vi "FgenChannelData2 FPCluster.vi"(8 "error in (no error)":errorcluster, 10 "Channel Index":i32, 11 "CS++FgenChannelData in":refnum<class "CS++FgenChannelData.lvclass">) -> (0 "error out":errorcluster, 1 "FM-Modulation":cluster{"Enabled":bool, "Source":i32}={"Enabled"=TRUE, "Source"=0} {"Source" items=["Internal", "External"]}, 2 "AM-Modulation":cluster{"Enabled":bool, "Source":i32}={"Enabled"=TRUE, "Source"=0} {"Source" items=["Internal", "External"]}, 3 "Standard-Waveform":T2={"Enabled"=TRUE, "Operation Mode"=0, "Impedance"=50.0, "Waveform"=1, "Frequency"=1000.0, "Amplitude"=1.0, "DC Offset"=0.0, "Trigger Source"=1, "Burst Count"=1, "Start Phase"=0.0, "Set/Single"=FALSE} {"Start Phase" format="%.3f"; "Trigger Source" items=["Internal"=3, "External"=1, "Software Trigger Function"=2, "PXI TRIG0 or VXI TTL0"=111, "PXI TRIG1 or VXI TTL1"=112, "PXI TRIG2 or VXI TTL2"=113, "PXI TRIG3 or VXI TTL3"=114, "PXI TRIG4 or VXI TTL4"=115, "PXI TRIG5 or VXI TTL5"=116, "PXI TRIG6 or VXI TTL6"=117, "PXI TRIG7 or VXI TTL7"=118, "ECL0"=119, "ECL1"=120, "PXI Star"=131, "RTSI 0"=141, "RTSI 1"=142, "RTSI 2"=143, "RTSI 3"=144, "RTSI 4"=145, "RTSI 5"=146, "RTSI 6"=147]; "Frequency" format="%^.3e"; "DC Offset" format="%.3f"; "Amplitude" format="%.3f"; "Waveform" items=["Sine"=1, "Square"=2, "Triangle"=3, "Ramp Up"=4, "Ramp Down"=5, "DC"=6]; "Impedance" format="%.3f"; "Operation Mode" items=["Continuous", "Burst"]}, 4 "Advanced Trigger":T1 {"Trigger Slope)" items=["Positive", "Negative", "Either"]}, 5 "Resume Trigger":T1 {"Trigger Slope)" items=["Positive", "Negative", "Either"]}, 6 "Stop Trigger":T1 {"Trigger Slope)" items=["Positive", "Negative", "Either"]}, 7 "Start Trigger":T1 {"Trigger Slope)" items=["Positive", "Negative", "Either"]})   [LabVIEW 2013, in "CS++FgenGui.lvlib" / "CS++FgenGui.lvclass"]
doc: "This VI read channel data from object and writes it into FP cluster."
uses:
  CS++FgenGui.lvclass
  CS++FgenChannelData/CS++FgenChannelData.lvclass
  CS++FgenChannelData/CS++FgenChannelData.lvclass/CS++FgenChannelData.ctl
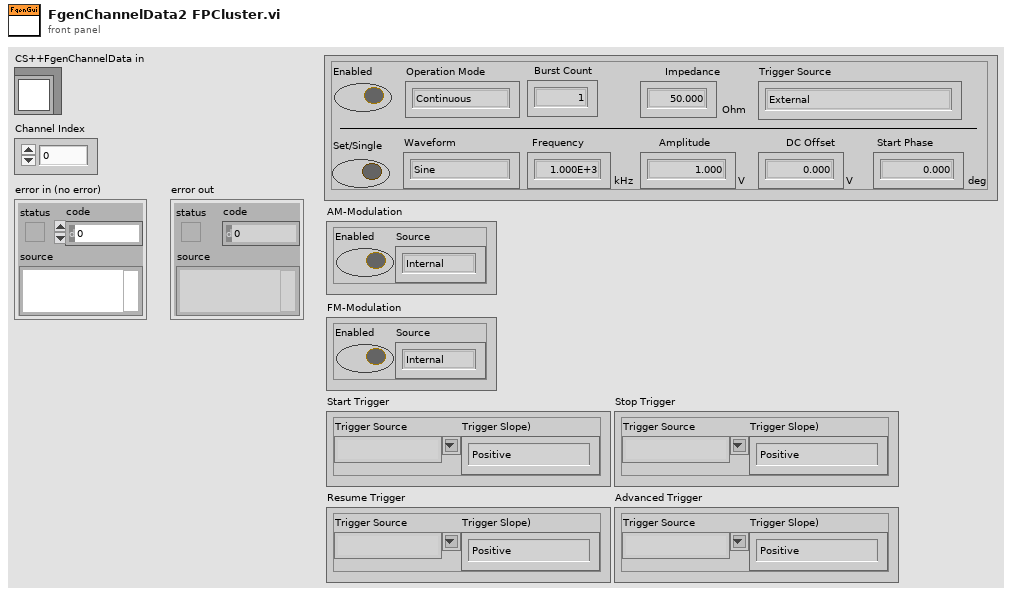
[diagram p1: front panel]
types:
  T1 = cluster{"Trigger Source":string, "Trigger Slope)":i32}
  T2 = cluster{"Enabled":bool, "Operation Mode":i32, "Impedance":dbl[unit], "Waveform":i32, "Frequency":dbl[unit], "Amplitude":dbl[unit], "DC Offset":dbl[unit], "Trigger Source":i32, "Burst Count":i32, "Start Phase":dbl[unit], "Set/Single":bool}
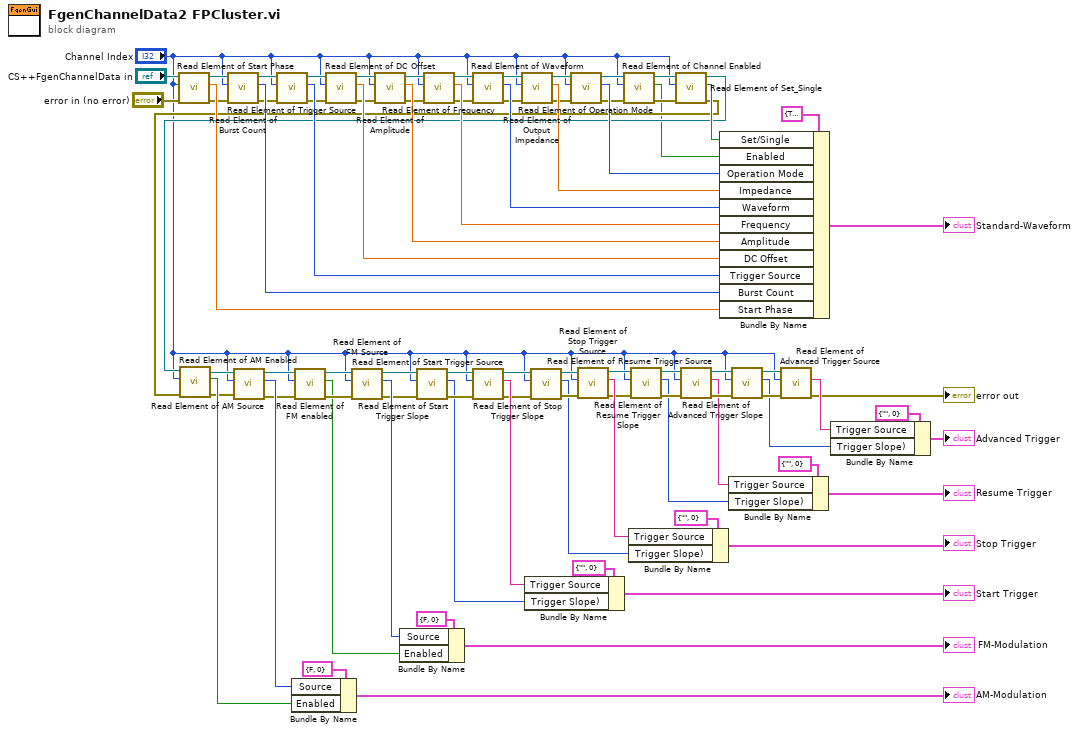
[diagram p0: block diagram]
diagram:
  n1 = call "Read Element of Start Phase.vi"("error in (no error)"="error in (no error)", "index"="Channel Index", "CS++FgenChannelData in"="CS++FgenChannelData in") -> ("error out"=w61:errorcluster, "start phase (0.00 Degrees)"=w71:dbl[unit], "CS++FgenChannelData out"=w69:refnum<class "CS++FgenChannelData.lvclass">)  [unwired: 6 in]
  n2 = call "Read Element of Burst Count.vi"("error in (no error)"=w61, "index"="Channel Index", "CS++FgenChannelData in"=w69) -> ("error out"=w62:errorcluster, "burst count (1)"=w72:i32, "CS++FgenChannelData out"=w70:refnum<class "CS++FgenChannelData.lvclass">)  [unwired: 6 in]
  n3 = call "Read Element of Trigger Source.vi"("error in (no error)"=w62, "index"="Channel Index", "CS++FgenChannelData in"=w70) -> ("error out"=w63:errorcluster, "trigger source (External)"=w73:i32, "CS++FgenChannelData out"=w74:refnum<class "CS++FgenChannelData.lvclass">)  [unwired: 6 in]
  n4 = call "Read Element of DC Offset.vi"("error in (no error)"=w63, "index"="Channel Index", "CS++FgenChannelData in"=w74) -> ("error out"=w64:errorcluster, "dc offset (0.00 V)"=w76:dbl[unit], "CS++FgenChannelData out"=w75:refnum<class "CS++FgenChannelData.lvclass">)  [unwired: 6 in]
  n5 = call "Read Element of Amplitude.vi"("error in (no error)"=w64, "index"="Channel Index", "CS++FgenChannelData in"=w75) -> ("error out"=w65:errorcluster, "amplitude (1.00 V)"=w77:dbl[unit], "CS++FgenChannelData out"=w78:refnum<class "CS++FgenChannelData.lvclass">)  [unwired: 6 in]
  n6 = call "Read Element of Frequency.vi"("error in (no error)"=w65, "index"="Channel Index", "CS++FgenChannelData in"=w78) -> ("error out"=w66:errorcluster, "frequency (1000.0 Hz)"=w79:dbl[unit], "CS++FgenChannelData out"=w80:refnum<class "CS++FgenChannelData.lvclass">)  [unwired: 6 in]
  n7 = call "Read Element of Waveform.vi"("error in (no error)"=w66, "index"="Channel Index", "CS++FgenChannelData in"=w80) -> ("error out"=w67:errorcluster, "waveform (Sine)"=w81:i32, "CS++FgenChannelData out"=w82:refnum<class "CS++FgenChannelData.lvclass">)  [unwired: 6 in]
  n8 = call "Read Element of Output Impedance.vi"("error in (no error)"=w67, "index"="Channel Index", "CS++FgenChannelData in"=w82) -> ("error out"=w68:errorcluster, "impedance (50 Ohms)"=w83:dbl[unit], "CS++FgenChannelData out"=w84:refnum<class "CS++FgenChannelData.lvclass">)  [unwired: 6 in]
  n9 = call "Read Element of Operation Mode.vi"("error in (no error)"=w68, "index"="Channel Index", "CS++FgenChannelData in"=w84) -> ("error out"=w4:errorcluster, "operation mode (Continuous)"=w85:i32, "CS++FgenChannelData out"=w6:refnum<class "CS++FgenChannelData.lvclass">)  [unwired: 6 in]
  n10 = call "Read Element of Channel Enabled.vi"("error in (no error)"=w4, "index"="Channel Index", "CS++FgenChannelData in"=w6) -> ("error out"=w2:errorcluster, "channel enabled (True)"=w1:bool, "CS++FgenChannelData out"=w5:refnum<class "CS++FgenChannelData.lvclass">)  [unwired: 6 in]
  n11 = call "Read Element of Set_Single.vi"("error in (no error)"=w2, "index"="Channel Index", "CS++FgenChannelData in"=w5) -> ("error out"=w8:errorcluster, "Set/Single"=w9:bool, "CS++FgenChannelData out"=w7:refnum<class "CS++FgenChannelData.lvclass">)  [unwired: 6 in]
  n12 = call "Read Element of AM Enabled.vi"("error in (no error)"=w8, "index"="Channel Index", "CS++FgenChannelData in"=w7) -> ("error out"=w54:errorcluster, "AM enabled (True)"=w57:bool, "CS++FgenChannelData out"=w55:refnum<class "CS++FgenChannelData.lvclass">)  [unwired: 6 in]
  n13 = call "Read Element of AM Source.vi"("error in (no error)"=w54, "index"="Channel Index", "CS++FgenChannelData in"=w55) -> ("error out"=w49:errorcluster, "source (Internal)"=w56:i32, "CS++FgenChannelData out"=w52:refnum<class "CS++FgenChannelData.lvclass">)  [unwired: 6 in]
  n14 = Bundle By Name(cluster=cluster{"Enabled":bool, "Source":i32} {"Enabled"=FALSE, "Source"=0} ("AM-Modulation"), "Source"=w56, "Enabled"=w57) -> (→"AM-Modulation":cluster{"Enabled":bool, "Source":i32})
  n15 = call "Read Element of FM enabled.vi"("error in (no error)"=w49, "index"="Channel Index", "CS++FgenChannelData in"=w52) -> ("error out"=w50:errorcluster, "FM enabled (True)"=w48:bool, "CS++FgenChannelData out"=w51:refnum<class "CS++FgenChannelData.lvclass">)  [unwired: 6 in]
  n16 = call "Read Element of FM Source.vi"("error in (no error)"=w50, "index"="Channel Index", "CS++FgenChannelData in"=w51) -> ("error out"=w43:errorcluster, "source (Internal)"=w47:i32, "CS++FgenChannelData out"=w44:refnum<class "CS++FgenChannelData.lvclass">)  [unwired: 6 in]
  n17 = Bundle By Name(cluster=cluster{"Enabled":bool, "Source":i32} {"Enabled"=FALSE, "Source"=0} ("FM-Modulation"), "Source"=w47, "Enabled"=w48) -> (→"FM-Modulation":cluster{"Enabled":bool, "Source":i32})
  n18 = call "Read Element of Start Trigger Slope.vi"("error in (no error)"=w43, "index"="Channel Index", "CS++FgenChannelData in"=w44) -> ("error out"=w41:errorcluster, "Trigger Slope (Positive)"=w40:i32, "CS++FgenChannelData out"=w42:refnum<class "CS++FgenChannelData.lvclass">)  [unwired: 6 in]
  n19 = call "Read Element of Start Trigger Source.vi"("error in (no error)"=w41, "index"="Channel Index", "CS++FgenChannelData in"=w42) -> ("error out"=w35:errorcluster, "Trigger Source (None)"=w38:string, "CS++FgenChannelData out"=w36:refnum<class "CS++FgenChannelData.lvclass">)  [unwired: 6 in]
  n20 = Bundle By Name(cluster=T1 {"Trigger Source"="", "Trigger Slope)"=0} ("Start Trigger"), "Trigger Source"=w38, "Trigger Slope)"=w40) -> (→"Start Trigger":T1)
  n21 = call "Read Element of Stop Trigger Slope.vi"("error in (no error)"=w35, "index"="Channel Index", "CS++FgenChannelData in"=w36) -> ("error out"=w33:errorcluster, "Trigger Slope (Positive)"=w31:i32, "CS++FgenChannelData out"=w34:refnum<class "CS++FgenChannelData.lvclass">)  [unwired: 6 in]
  n22 = call "Read Element of Stop Trigger Source.vi"("error in (no error)"=w33, "index"="Channel Index", "CS++FgenChannelData in"=w34) -> ("error out"=w27:errorcluster, "Trigger Source (None)"=w30:string, "CS++FgenChannelData out"=w28:refnum<class "CS++FgenChannelData.lvclass">)  [unwired: 6 in]
  n23 = Bundle By Name(cluster=T1 {"Trigger Source"="", "Trigger Slope)"=0} ("Stop Trigger"), "Trigger Source"=w30, "Trigger Slope)"=w31) -> (→"Stop Trigger":T1)
  n24 = call "Read Element of Resume Trigger Slope.vi"("error in (no error)"=w27, "index"="Channel Index", "CS++FgenChannelData in"=w28) -> ("error out"=w25:errorcluster, "Trigger Slope (Positive)"=w18:i32, "CS++FgenChannelData out"=w26:refnum<class "CS++FgenChannelData.lvclass">)  [unwired: 6 in]
  n25 = call "Read Element of Resume Trigger Source.vi"("error in (no error)"=w25, "index"="Channel Index", "CS++FgenChannelData in"=w26) -> ("error out"=w23:errorcluster, "Trigger Source (None)"=w19:string, "CS++FgenChannelData out"=w24:refnum<class "CS++FgenChannelData.lvclass">)  [unwired: 6 in]
  n26 = Bundle By Name(cluster=T2 {"Enabled"=TRUE, "Operation Mode"=0, "Impedance"=50.0, "Waveform"=1, "Frequency"=1000.0, "Amplitude"=1.0, "DC Offset"=0.0, "Trigger Source"=1, "Burst Count"=1, "Start Phase"=0.0, "Set/Single"=FALSE} ("Standard-Waveform"), "Set/Single"=w9, "Enabled"=w1, "Operation Mode"=w85, "Impedance"=w83, "Waveform"=w81, "Frequency"=w79, "Amplitude"=w77, "DC Offset"=w76, "Trigger Source"=w73, "Burst Count"=w72, "Start Phase"=w71) -> (→"Standard-Waveform":T2)
  n27 = Bundle By Name(cluster=T1 {"Trigger Source"="", "Trigger Slope)"=0} ("Resume Trigger"), "Trigger Source"=w19, "Trigger Slope)"=w18) -> (→"Resume Trigger":T1)
  n28 = call "Read Element of Advanced Trigger Slope.vi"("error in (no error)"=w23, "index"="Channel Index", "CS++FgenChannelData in"=w24) -> ("error out"=w22:errorcluster, "Trigger Slope (Positive)"=w13:i32, "CS++FgenChannelData out"=w21:refnum<class "CS++FgenChannelData.lvclass">)  [unwired: 6 in]
  n29 = call "Read Element of Advanced Trigger Source.vi"("error in (no error)"=w22, "index"="Channel Index", "CS++FgenChannelData in"=w21) -> ("error out"=→"error out":errorcluster, "Trigger Source (None)"=w14:string)  [unwired: 6 in, 1 out]
  n30 = Bundle By Name(cluster=T1 {"Trigger Source"="", "Trigger Slope)"=0} ("Advanced Trigger"), "Trigger Source"=w14, "Trigger Slope)"=w13) -> (→"Advanced Trigger":T1)
